vi "shutdown_splash.vi"() -> ()   [LabVIEW 2018]
panel:
  out "Shutting Down TimeTagger":u8(slide) scale=0.0..100.0
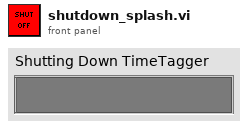
[diagram p1: front panel]
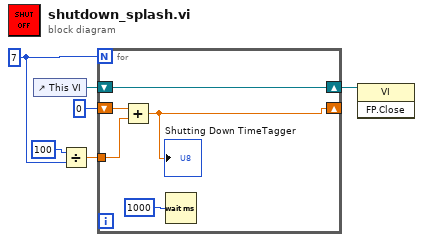
[diagram p0: block diagram]
diagram:
  w6 = 7
  n1 = control-ref of="This VI"() -> (w2:refnum<vi>)
  n2 = Divide(x=100, y=w6) -> (x/y=w5:dbl)
  n3 = for {
    N: w6 -> [_]
    tunnel: w5 -> [w9]
    shift-right: [w8] -> _
    shift-left: 0 -> [w10]
    shift-right: [w7] -> w1
    shift-left: w2 -> [w7]
    n4 = Add(x=w10, y=w9) -> (x+y=w8:dbl)
    "Shutting Down TimeTagger" <- w8
    n5 = Wait (ms)(milliseconds to wait=u32 1000) -> ()  [unwired: 1 out]
  }
  n6 = invoke class="VI" method="FP.Close"(reference=w1) -> ()  [unwired: 2 in, 3 out]
